vi "Localized Strings.vi"() -> ()   [LabVIEW 2020, in "Message Maker Provider.lvlib"]
uses:
  Message Maker Provider.lvlib
panel:
  in  "Are you sure?":string="Are you sure?"
  in  "Are you sure about making abstract message?":string="Abstract messages were a mechanism for making nested actors not be hardcoded to only talk to a particular type of caller actor prior to the introduction of interfaces. Interfaces were introduced in LabVIEW 2020 to offer a dramatically easier way to break dependencies between actors.\n\nContinue creating an abstract message?"
  in  "Select the reference method":string="Select the reference method:"
  in  "Create Messages for Actors":string="Create Messages for Actors"
  in  "Create Abstract Message for Caller":string="Create Abstract Message for Caller"
  in  "Create Messages for Actor":string="Create Messages for Actor"
  in  "Create Messages":string="Create Actor Messages"
  in  "Create Child of Abstract Message":string="Create Child of Abstract Message"
  in  "Create Message":string="Create Message"
  in  "Actor Framework":string="Actor Framework"
  in  "Select the parent abstract message":string="Select the parent abstract message:"
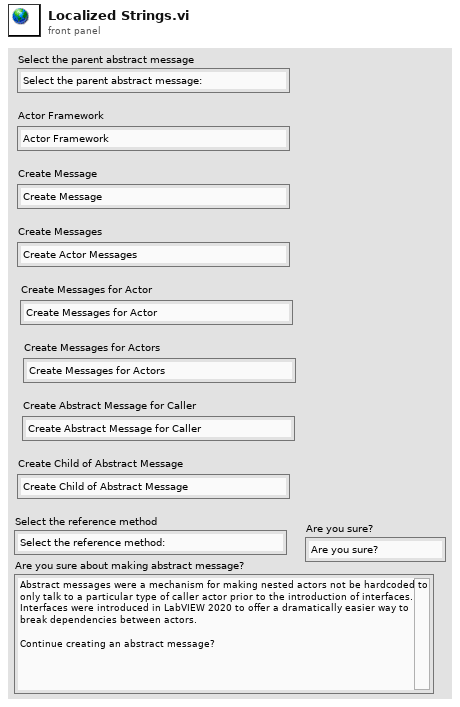
[diagram p1: front panel]
diagram:
